vi "Spectrum using Chirp Z Transform.vi"() -> ()   [LabVIEW 2020]
doc: "This example demonstrates how to use the Chirp Z Transform VI to evaluate a partial DFT. Also, it shows how to calculate the starting point and increment for the Chirp Z Transform VI giving the sampling frequency, high frequency, low frequency and number of bins."
uses:
  <vilib>/Analysis/2dsp.llb/Chirp Z Transform (DBL).vi
  <vilib>/Analysis/2dsp.llb/Real FFT.vi
  <vilib>/Analysis/NI_AALPro.lvlib
  <vilib>/Analysis/NI_AALBase.lvlib
panel:
  in  "Stop":bool
  in  "f2 (Hz)":dbl(slide)=60.0 scale=50.0..70.0
  in  "f1 (Hz)":dbl(slide)=55.0 scale=40.0..60.0
  out "Signal Waveform":waveform(dbl)(graph)
  out "Amplitude Spectrum":cluster{"high freq. (Hz)":dbl, dbl, dbl[]}[](graph)
  in  "# of bins for Chirp Z Transform":i32=16
  in  "high frequency (Hz)":dbl=65.0
  in  "low frequency (Hz)":dbl=50.0
  in  "fs (Hz)":dbl=1000.0
  # "Overview: Demonstrates how to use the Chirp Z Transform VI to evaluate a partial Discrete Fourier Transform (DFT).\nRequirement: LabVIEW Full Development System\nInstructions:\n1. Run the VI. Notice that if the # of bins is equal to the FFT bins in the range of [low freq, high freq], the Chirp Z transform result is the same as that of FFT. Here the VI performs a 1000-point FFT on a signal with 1000 Hz sampling frequency. So in the frequency range [50Hz, 65Hz], there are 16 FFT bins.\n2. Set # of bins for Chirp Z Transform to 16. The Chirp Z Transform VI returns the same result as that of FFT in the range [50Hz, 65Hz].\n3. Click Stop to stop the VI."
  # "Signal Settings"
  # "Spectrum Settings"
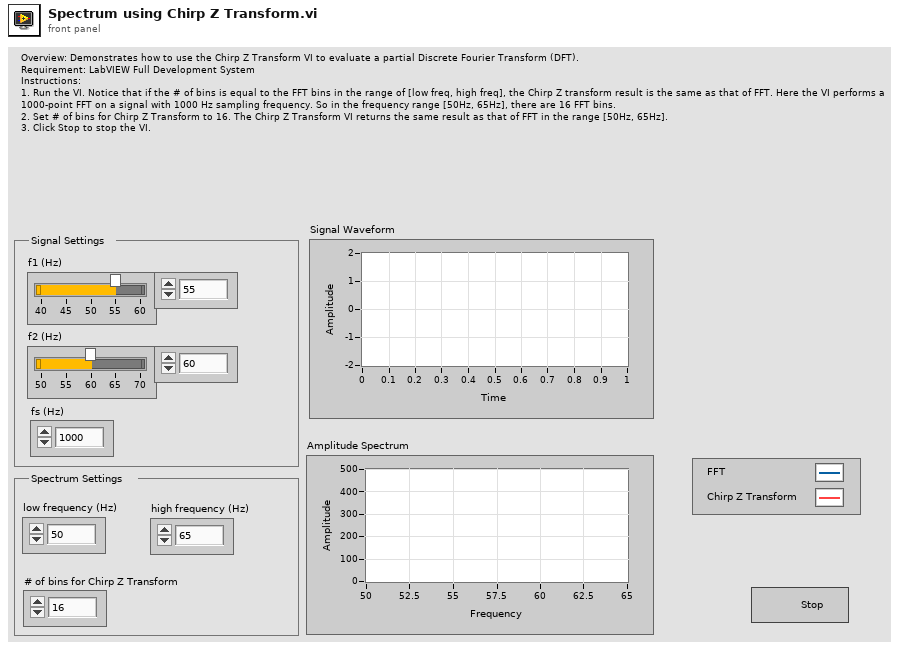
[diagram p1: front panel]
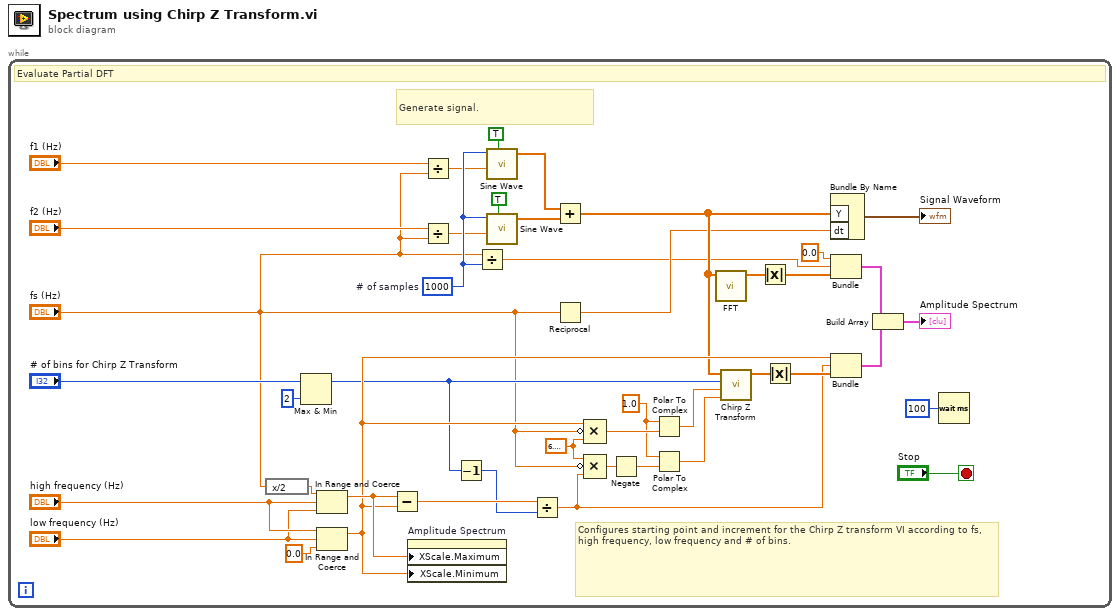
[diagram p0: block diagram]
diagram:
  n1 = while {
    stop <- "Stop" stop-if-true
    w4 = 1.0
    w16 = 6.283185307179586
    w30 = 1000  # # of samples
    # "Configures starting point and increment for the Chirp Z transform VI according to fs, high frequency, low frequency and # of bins."
    # "Generate signal."
    # "Evaluate Partial DFT"
    n2 = expression code="x/2"("fs (Hz)") -> (w14:dbl)
    n3 = Max & Min(x="# of bins for Chirp Z Transform", y=2) -> (max(x,y)=w28:i32)  [unwired: 1 out]
    n4 = In Range and Coerce(upper limit=w14, x="high frequency (Hz)", lower limit="low frequency (Hz)") -> (coerced(x)=w35:dbl)  [unwired: 1 out]
    n5 = In Range and Coerce(upper limit="high frequency (Hz)", x="low frequency (Hz)", lower limit=0.0) -> (coerced(x)=w33:dbl)  [unwired: 1 out]
    n6 = Subtract(x=w35, y=w33) -> (x-y=w27:dbl)
    n7 = property on="Amplitude Spectrum" class="WFGraph (strict)"("XScale.Maximum"=w35, "XScale.Minimum"=w33) -> ()  [unwired: 2 in, 2 out]
    n8 = Divide(x="f1 (Hz)", y="fs (Hz)") -> (x/y=w23:dbl)
    n9 = Divide(x="f2 (Hz)", y="fs (Hz)") -> (x/y=w20:dbl)
    n10 = Decrement(x=w28) -> (x-1=w12:i32)
    n11 = Divide(x="fs (Hz)", y=w30) -> (x/y=w10:dbl)
    n12 = call <vilib>:"Sine Wave.vi"("samples"=w30, "frequency"=w23, "reset phase"=TRUE) -> ("sine wave"=w21:dbl[])  [unwired: 2 in, 2 out]
    n13 = call <vilib>:"Sine Wave.vi"("samples"=w30, "frequency"=w20, "reset phase"=TRUE) -> ("sine wave"=w19:dbl[])  [unwired: 2 in, 2 out]
    n14 = Divide(x=w27, y=w12) -> (x/y=w2:dbl)
    n15 = Add(x=w21, y=w19) -> (x+y=w25:dbl[])
    n16 = Reciprocal(x="fs (Hz)") -> (1/x=w17:dbl)
    n17 = Compound Arithmetic op=MULTIPLY(w33, invert "fs (Hz)", w16) -> (w8:dbl)
    n18 = Compound Arithmetic op=MULTIPLY(w16, invert "fs (Hz)", w2) -> (w6:dbl)
    n19 = Negate(x=w6) -> (-x=w3:dbl)
    n20 = Polar To Complex(1:w8, 2:w4) -> (0:w7:cdb)
    n21 = Polar To Complex(1:w3, 2:w4) -> (0:w5:cdb)
    n22 = call-poly <vilib>:"FFT.vi"("X"=w25) -> ("FFT {X}"=w43:cdb[])  [unwired: 2 in, 8 out]
    n23 = call-poly <vilib>:"Chirp Z Transform.vi"("increment"=w5, "starting point"=w7, "# of bins"=w28, "X"=w25) -> ("Chirp-Z {X}"=w42:cdb[])  [unwired: 1 in, 6 out]
    n24 = Absolute Value(x=w43) -> (abs(x)=w40:dbl[])
    n25 = Absolute Value(x=w42) -> (abs(x)=w39:dbl[])
    n26 = Bundle By Name("Y"=w25, "dt"=w17) -> (→"Signal Waveform":waveform(dbl))  [unwired: 1 out]
    n27 = Bundle(0.0, w10, w40) -> (w38:cluster{dbl, dbl, dbl[]})  [unwired: 1 out]
    n28 = Bundle("high frequency (Hz)"=w33, w2, w39) -> (w37:cluster{"high frequency (Hz)":dbl, dbl, dbl[]})  [unwired: 1 out]
    n29 = Build Array(w38, w37) -> (→"Amplitude Spectrum":cluster{"high frequency (Hz)":dbl, dbl, dbl[]}[])
    n30 = Wait (ms)(milliseconds to wait=u32 100) -> ()  [unwired: 1 out]
  }
